vi "Qn15_Z.vi"(11 "String":string) -> (3 "Qn":dbl[](array[numeric]))   [LabVIEW 2015]
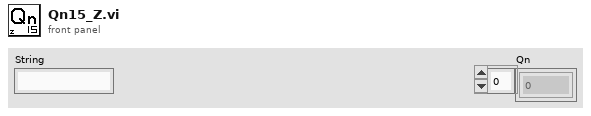
[diagram p1: front panel]
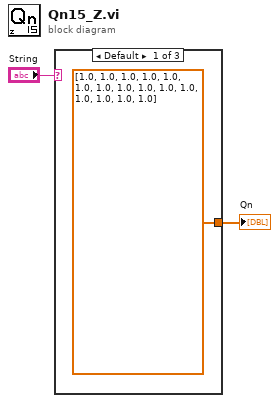
[diagram p0: block diagram]
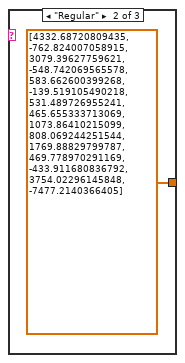
[diagram p2: hidden frame]
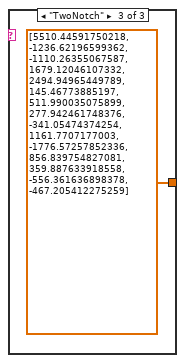
[diagram p3: hidden frame]
diagram:
  n1 = case shown="Default" "String" {
    tunnel: [dbl[] [1.0, 1.0, 1.0, 1.0, 1.0, 1.0, 1.0, 1.0, 1.0, 1.0, 1.0, 1.0, 1.0, 1.0, 1.0] ("Qn") dbl[] [4332.68720809435, -762.824007058915, 3079.39627759621, -548.742069565578, 583.662600399268, -139.519105490218, 531.489726955241, 465.655333713069, 1073.86410215099, 808.069244251544, 1769.88829799787, 469.778970291169, -433.911680836792, 3754.02296145848, -7477.2140366405] ("Qn") dbl[] [5510.44591750218, -1236.62196599362, -1110.26355067587, 1679.12046107332, 2494.94965449789, 145.46773885197, 511.990035075899, 277.942461748376, -341.05474374254, 1161.7707177003, -1776.57257852336, 856.839754827081, 359.887633918558, -556.361636898378, -467.205412275259] ("Qn")] -> w2
    frame Default {
    }
    frame "Regular" {
    }
    frame "TwoNotch" {
    }
  }
  "Qn" <- w2
